vi "dbscan.vi"   [LabVIEW 2012]
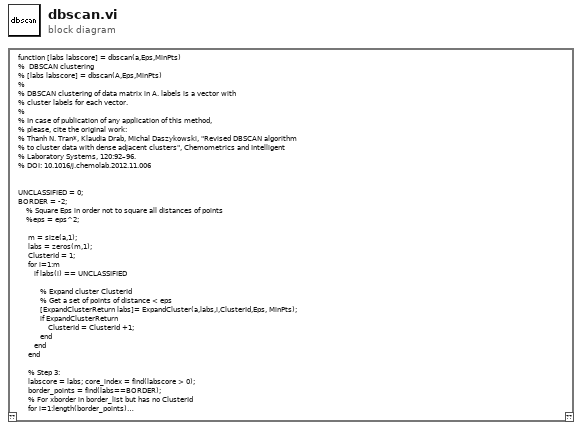
[diagram p0: block diagram]
diagram:
  n1 = mathscript code="function [labs labscore] = dbscan(a,Eps,MinPts)\n%  DBSCAN clustering\n% [labs labscore] = dbscan(A,Eps,MinPts)\n%\n% DBSCAN clustering of data matrix in A. labels is a vector with \n% cluster labels for each vector.\n% \n% In case of publication of any application of this method,\n% please, cite the original work:\n% Thanh N. Tran*, Klaudia Drab, Michal Daszykowski, \"Revised DBSCAN algorithm \n% to cluster data with dense adjacent clusters\", Chemometrics and Intelligent \n% Laboratory Systems, 120:92–96.\n% DOI: 10.1016/j.chemolab.2012.11.006 \n\n\nUNCLASSIFIED = 0;\nBORDER = -2;\n    % Square Eps in order not to square all distances of points\n    %eps = eps^2;\n    \n     m = size(a,1);\n     labs = zeros(m,1);\n     ClusterId = 1;\n     for i=1:m\n        if labs(i) == UNCLASSIFIED                 \n            \n           % Expand cluster ClusterId\n           % Get a set of points of distance < eps\n           [ExpandClusterReturn labs]= ExpandCluster(a,labs,i,ClusterId,Eps, MinPts);\n           if ExpandClusterReturn\n               ClusterId = ClusterId +1;\n           end\n        end\n     end\n\n     % Step 3:\n     labscore = labs; core_index = find(labscore > 0);\n     border_points = find(labs==BORDER);\n     % For xborder in border_list but has no ClusterId\n     for i=1:length(border_points)\n            % xborder in border_list\n            currentB = border_points(i);\n            d=distance(+a(currentB,:),+a(core_index,:),1);\n            % the closest core-points \n            [tmp nearest_core]=min(d);\n            nearest_core_index=core_index(nearest_core);\n            %Assign xborder to ClusterId of the closest core-points \n            labs(currentB)=labs(nearest_core_index);\n     end\nend"() -> ()  [unwired: 1 in, 1 out]
